vi "temperature Converter.vi"() -> ()   [LabVIEW 2014]
panel:
  in  "Temperature":dbl
  in  "Enum":T1(ring)
  out "Converted temperature":dbl
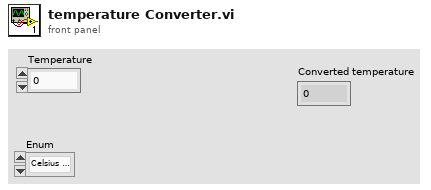
[diagram p1: front panel]
types:
  T1 = enum16{"Celsius to Fahrenheit", "Fahrenheit to Celsius", "Celsius to Kelvin", "Fahrenheit to Kelvin"}
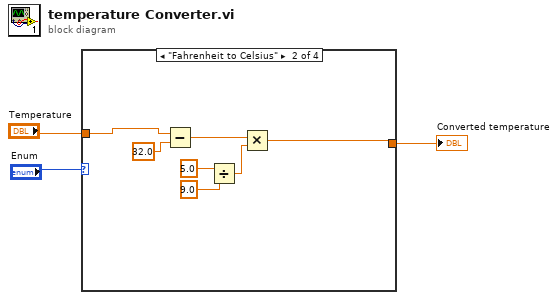
[diagram p0: block diagram]
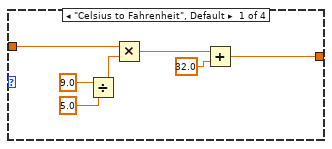
[diagram p2: hidden frame]
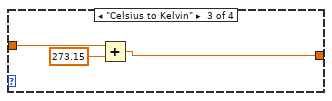
[diagram p3: hidden frame]
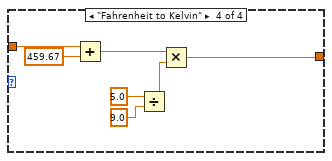
[diagram p4: hidden frame]
diagram:
  n1 = case shown="\"Fahrenheit to Celsius\"" "Enum" {
    tunnel: "Temperature" -> [w10 w11 w20 w27]
    tunnel: [w7 w15 w18 w21] -> w3
    frame "Celsius to Fahrenheit", Default {
      n2 = Divide(x=9.0, y=5.0) -> (x/y=w6:dbl)
      n3 = Multiply(x=w10, y=w6) -> (x*y=w9:dbl)
      n4 = Add(x=w9, y=32.0) -> (x+y=w7:dbl)
    }
    frame "Fahrenheit to Celsius" {
      n5 = Subtract(x=w11, y=32.0) -> (x-y=w16:dbl)
      n6 = Divide(x=5.0, y=9.0) -> (x/y=w14:dbl)
      n7 = Multiply(x=w16, y=w14) -> (x*y=w15:dbl)
    }
    frame "Celsius to Kelvin" {
      n8 = Add(x=w20, y=273.15) -> (x+y=w18:dbl)
    }
    frame "Fahrenheit to Kelvin" {
      n9 = Add(x=w27, y=459.67) -> (x+y=w25:dbl)
      n10 = Divide(x=5.0, y=9.0) -> (x/y=w22:dbl)
      n11 = Multiply(x=w25, y=w22) -> (x*y=w21:dbl)
    }
  }
  "Converted temperature" <- w3
